vi "Test Panel - Add test (SubVI).vi"(8 "error in":errorcluster) -> (0 "error Out":errorcluster, 1 "Station":string, 2 "Cancel?":bool, 3 "Test Plan":string)   [LabVIEW 2019]
uses:
  Controls/Add test-state.ctl
  Controls/eFGV States.ctl
  Controls/FGV States.ctl
panel:
  in  "Path":path
  out "Station Data":string[](array[string])
  out "Status out":string[](array[string])
  in  "Select Station":u16(ring) items=["Please Select...", "TEST", "CONSOL", "UCT", "ISO CONS", "SATURATION", "TRIAXIALSHEAR", "TEST UU"]
  out "Select Test Plan form the list :":u16(ring) items=["Please Select...", "1dconsol.gs", "a", "abc.gs", "bcheck50.gs", "consol test.gs", "consol400-100.gs", "load12N(Table).gs", "load192N(Table).gs", "load24N(Table).gs", "load384N(Table).gs", "load48N(Table).gs", "load6N(Table).gs", "load96N(Table).gs", "loading12N.gs", "loading200N.gs", "loading24N.gs", "loading400N.gs", "loading48N.gs", "loading96N.gs", "sada.gs", "Sat100-90.gs", "Sat200-190.gs", "Sat300-290.gs", "Sat400-390.gs", "Sat50-40.gs", "Shearbox.gs", "test UU.gs", "test.gs", "test1.gs", "triaxialshear.gs", "uctcompressiontest.gs", "unload24(Table).gs", "unload24.gs", "unload96(Table).gs", "unload96.gs"]
  in  "OK":bool
  in  "Cancel":bool
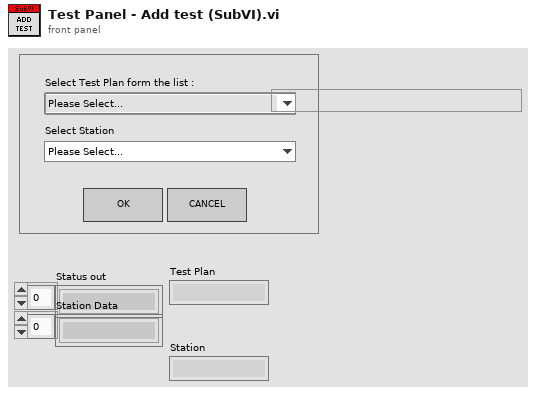
[diagram p1: front panel]
types:
  T1 = typedef "Add test-state.ctl" = enum16{"Init", "Idle", "Add", "Load Station", "Load", "Check Device", "Close", "Exit"}
  T2 = enum8{"Enabled", "Disabled", "Disabled and Grayed Out"}
  T3 = typedef "eFGV States.ctl" = enum16{"Init", "Read", "Write", "Exit"}
  T4 = typedef "FGV States.ctl" = enum16{"Read", "Write"}
  T5 = cluster{"TestPlan Section":string, "Key Value":string[]}[]
  T6 = cluster{"TestPlan Section":string, "Key Value":string[]}
  T7 = cluster{"Station Name":string, "Key Value":string[], "Key Names":string[]}[]
  T8 = cluster{"Station Name":string, "Key Value":string[], "Key Names":string[]}
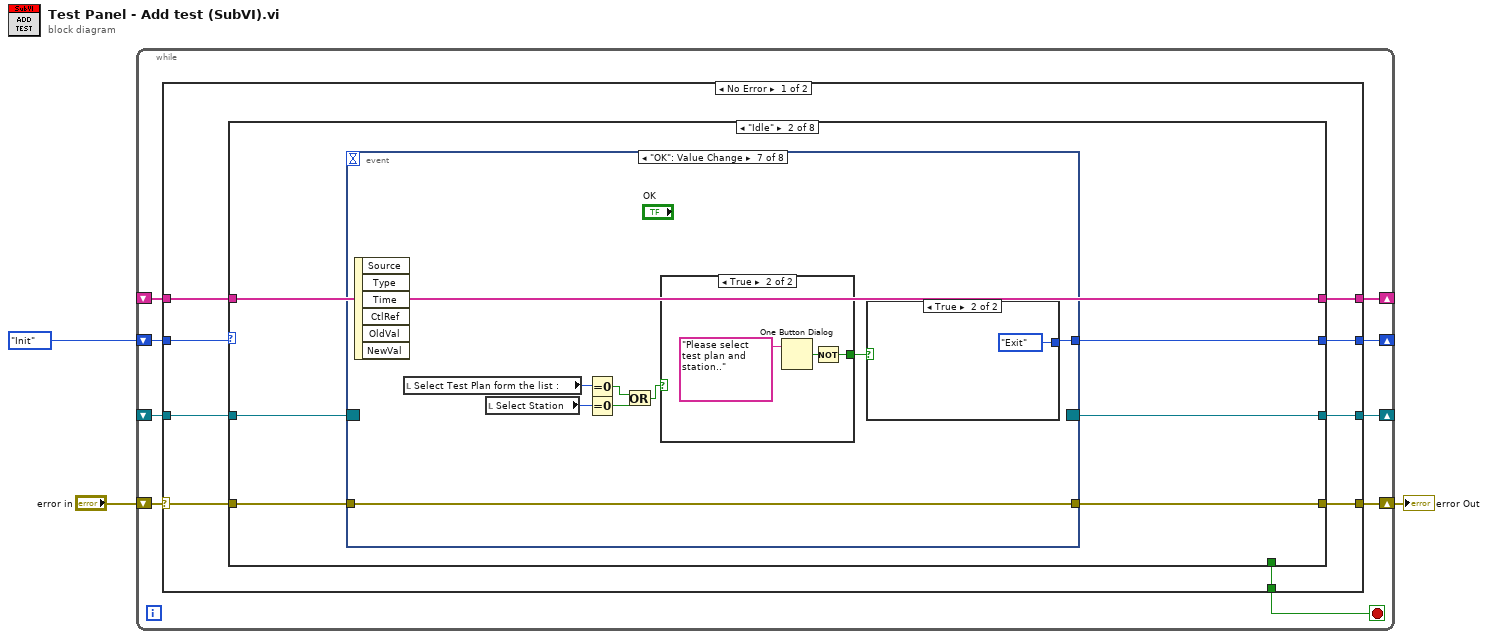
[diagram p0: block diagram]
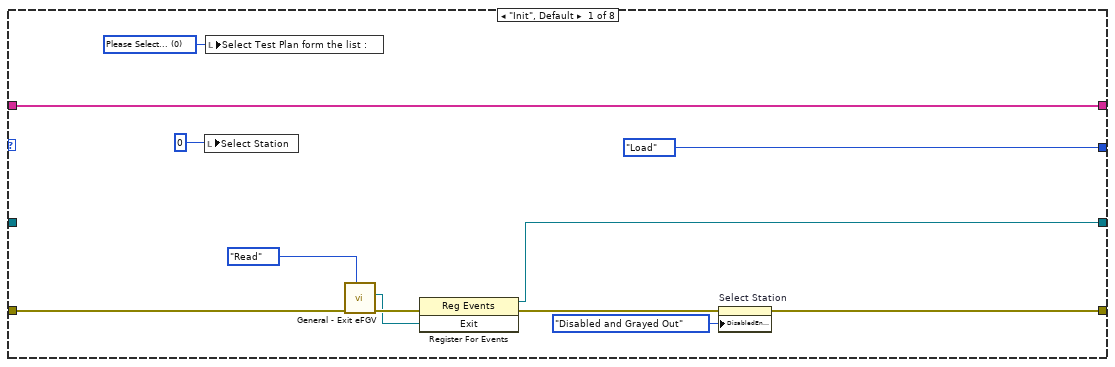
[diagram p2: hidden frame]
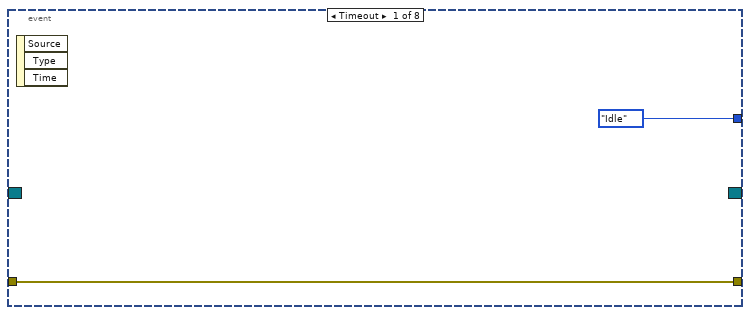
[diagram p3: hidden frame]
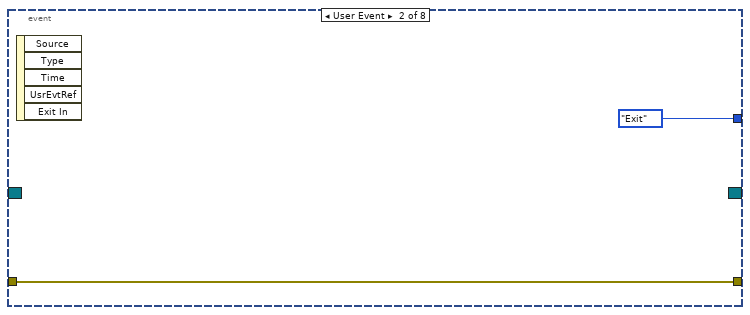
[diagram p4: hidden frame]
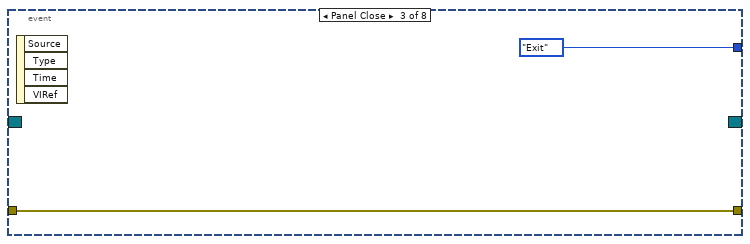
[diagram p5: hidden frame]
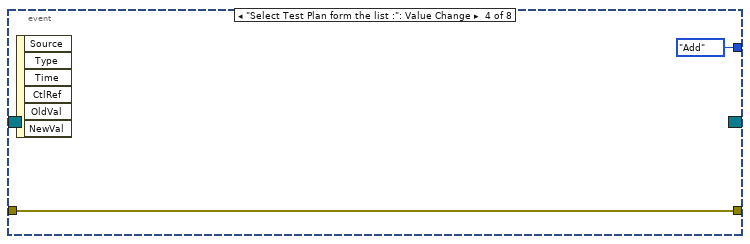
[diagram p6: hidden frame]
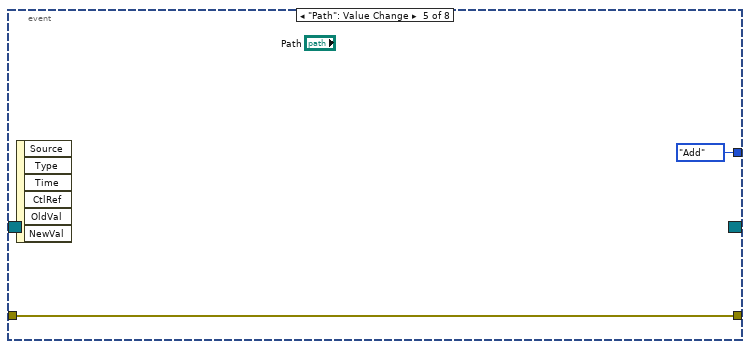
[diagram p7: hidden frame]
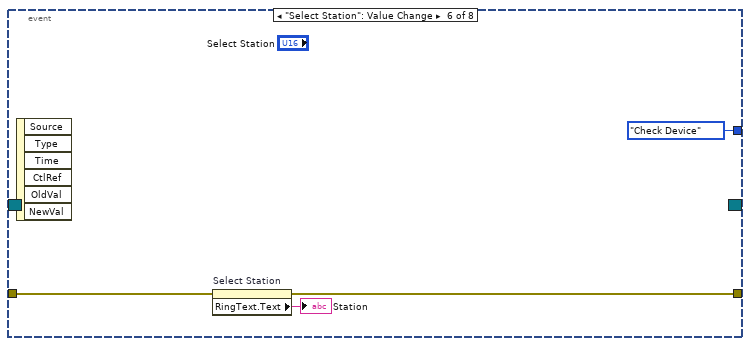
[diagram p8: hidden frame]
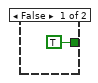
[diagram p9: hidden frame]
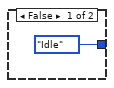
[diagram p10: hidden frame]
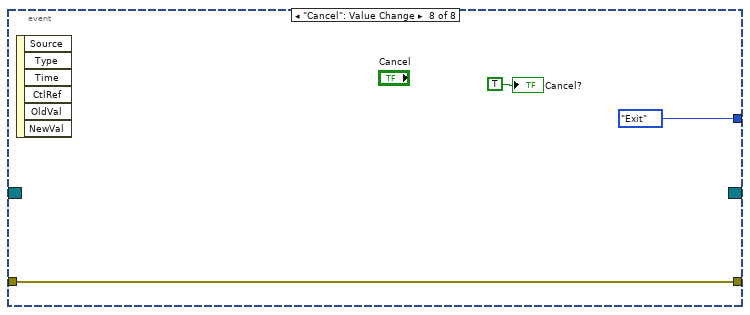
[diagram p11: hidden frame]
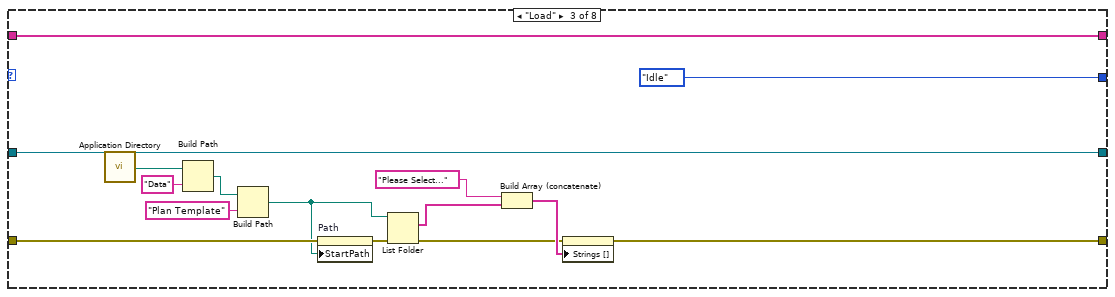
[diagram p12: hidden frame]
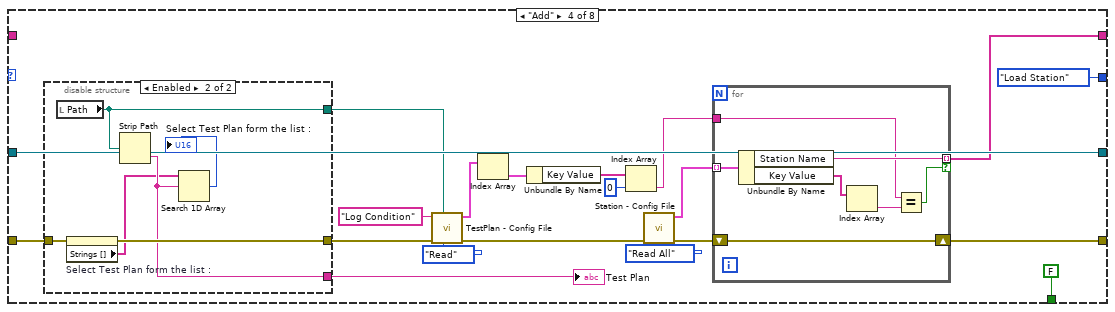
[diagram p13: hidden frame]
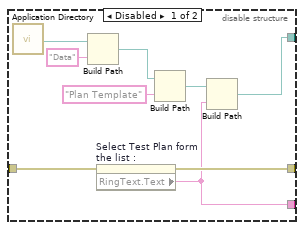
[diagram p14: hidden frame]
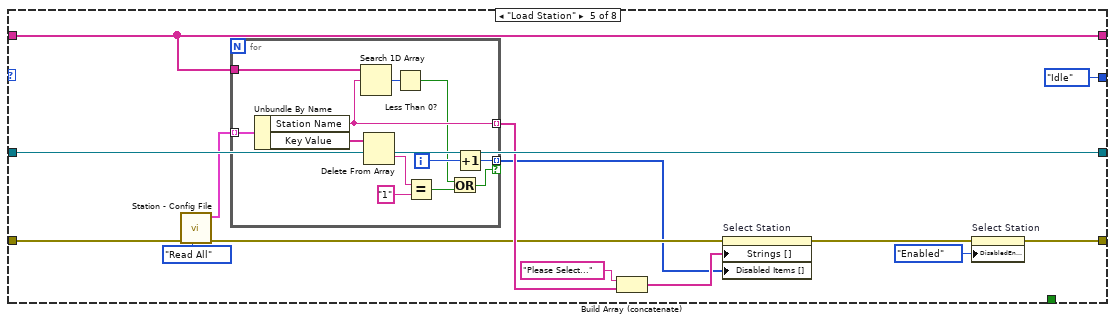
[diagram p15: hidden frame]
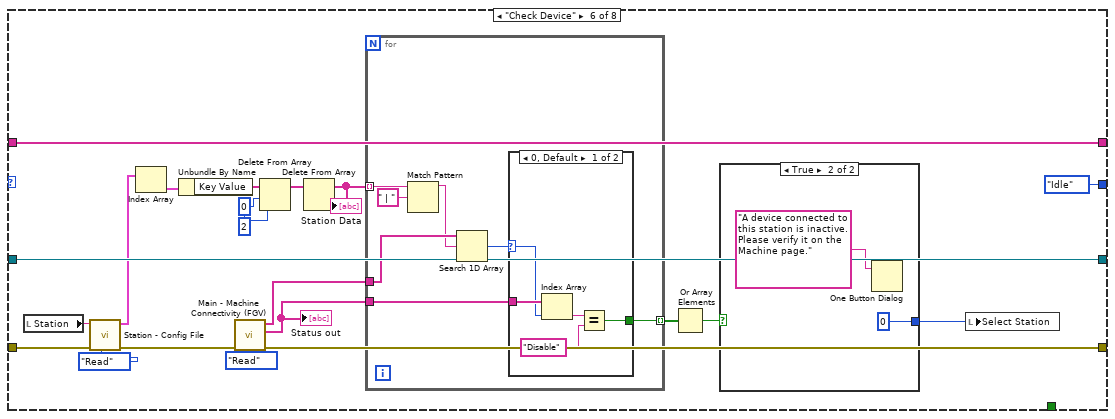
[diagram p16: hidden frame]
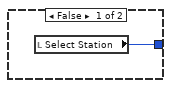
[diagram p17: hidden frame]
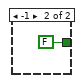
[diagram p18: hidden frame]
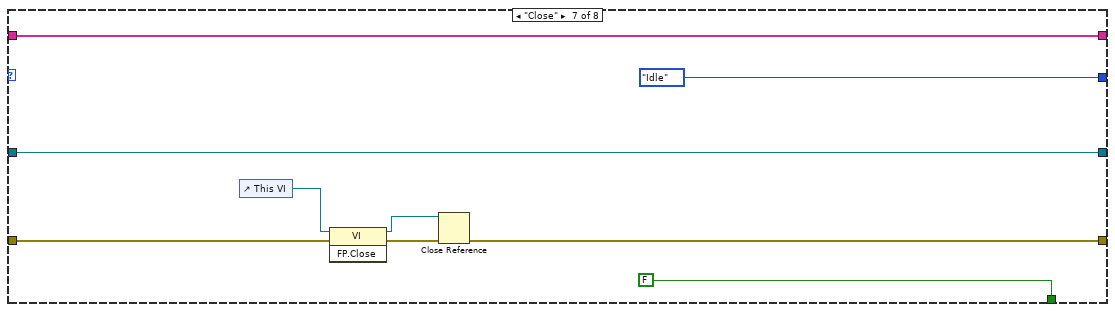
[diagram p19: hidden frame]
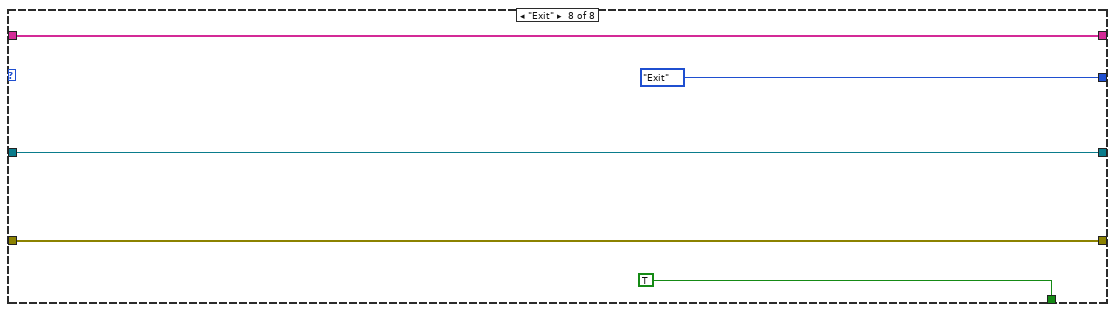
[diagram p20: hidden frame]
diagram:
  n1 = while {
    shift-right: [w11] -> w1
    shift-left: "error in" -> [w12]
    shift-right: [w9] -> _
    shift-left: Add_test-state."Init" -> [w10]
    shift-right: [w7] -> _
    shift-left: _ -> [w6]
    shift-right: [w5] -> _
    shift-left: _ -> [w4]
    stop <- w8 stop-if-true
    n2 = case shown="No Error" w12 {
      selector: w12 -> [w21 w210]
      tunnel: [w20 w208] -> w11
      tunnel: w10 -> [w19 _]
      tunnel: [w18 Add_test-state."Idle"] -> w9
      tunnel: [w17 _] -> w8
      tunnel: [w16 w209] -> w7
      tunnel: w6 -> [w15 w209]
      tunnel: [w14 w205] -> w5
      tunnel: w4 -> [w13 w205]
      frame No Error {
        n3 = case shown="\"Idle\"" w19 {
          tunnel: w21 -> [w29 w39 w72 w102 w136 w161 w195 w204]
          tunnel: [w24 w38 w74 w89 w128 w162 w193 w204] -> w20
          tunnel: [Add_test-state."Load" w37 Add_test-state."Idle" Add_test-state."Load Station" Add_test-state."Idle" Add_test-state."Idle" Add_test-state."Idle" Add_test-state."Exit"] -> w18
          tunnel: [_ _ _ FALSE _ _ FALSE TRUE] -> w17
          tunnel: [w30 w35 w85 w103 w141 w174 w199 w203] -> w16
          tunnel: w15 -> [_ w36 w85 w103 w141 w174 w199 w203]
          tunnel: [w26 w34 w75 w87 w131 w173 w191 w200] -> w14
          tunnel: w13 -> [w26 w34 w75 _ w131 w173 w191 w200]
          frame "Init", Default {
            w27 = u16 0 items=["Please Select..."] ("Select Test Plan form the list :")
            n4 = local write "Select Station"(0) -> ()
            n5 = local write "Select Test Plan form the list :"(w27) -> ()
            n6 = call "General - Exit eFGV.vi"("eFGV States"=eFGV_States."Read", "error in (no error)"=w29) -> ("error out"=w32:errorcluster, "Exit"=w31:refnum<user-event>)  [unwired: 7 in, 1 out]
            n7 = register-events(error in=w32, w31) -> (reference out=w30:refnum<event-registration>, error out=w25:errorcluster)  [unwired: 1 in]
            n8 = property on="Select Station" class="Ring (strict)"(error in=w25, "DisabledEnum"=T2."Disabled and Grayed Out" ("Disabled")) -> (error out=w24:errorcluster)  [unwired: 1 in, 1 out]
          }
          frame "Idle" {
            n9 = event shown="[6] \"OK\": Value Change" {
              selector: w36 -> [_ _ _ _ _ _ _ _]
              dyn-events: [_ _ _ _ _ _ _ _] -> w35
              timeout: _ -> [_ _ _ _ _ _ _ _]
              tunnel: w39 -> [w41 w43 w45 w47 w49 w51 w61 w69]
              tunnel: [w41 w43 w45 w47 w49 w52 w61 w69] -> w38
              tunnel: [Add_test-state."Idle" Add_test-state."Exit" Add_test-state."Exit" Add_test-state."Add" Add_test-state."Add" Add_test-state."Check Device" w59 Add_test-state."Exit"] -> w37
              event Timeout {
                n10 = event-data() -> ()  [unwired: 1 in, 3 out]
              }
              event User Event {
                n11 = event-data() -> ()  [unwired: 1 in, 5 out]
              }
              event Panel Close {
                n12 = event-data() -> ()  [unwired: 1 in, 4 out]
              }
              event "Select Test Plan form the list :": Value Change {
                n13 = event-data() -> ()  [unwired: 1 in, 6 out]
              }
              event "Path": Value Change {
                n14 = event-data() -> ()  [unwired: 1 in, 6 out]
              }
              event "Select Station": Value Change {
                n15 = event-data() -> ()  [unwired: 1 in, 6 out]
                n16 = property on="Select Station" class="Ring (strict)"(error in=w51) -> (error out=w52:errorcluster, "RingText.Text"=→"Station":string)  [unwired: 1 in, 1 out]
              }
              event "OK": Value Change {
                n17 = event-data() -> ()  [unwired: 1 in, 6 out]
                n18 = local read "Select Test Plan form the list :"() -> (w58:u16)
                n19 = local read "Select Station"() -> (w57:u16)
                n20 = Equal To 0?(x=w58) -> (x = 0?=w56:bool)
                n21 = Equal To 0?(x=w57) -> (x = 0?=w55:bool)
                n22 = Or(x=w56, y=w55) -> (x .or. y?=w54:bool)
                n23 = case shown="True" w54 {
                  tunnel: [TRUE w64] -> w60
                  frame False {
                  }
                  frame True {
                    n24 = One Button Dialog(message="Please select test plan and station..") -> (true=w65:bool)  [unwired: 1 in]
                    n25 = Not(x=w65) -> (.not. x?=w64:bool)
                  }
                }
                n26 = case shown="True" w60 {
                  tunnel: [Add_test-state."Idle" Add_test-state."Exit"] -> w59
                  frame False {
                  }
                  frame True {
                  }
                }
              }
              event "Cancel": Value Change {
                n27 = event-data() -> ()  [unwired: 1 in, 6 out]
                "Cancel?" <- TRUE
              }
            }
          }
          frame "Load" {
            n28 = call <vilib>:"Application Directory.vi"() -> ("Application Directory"=w77:path)
            n29 = Build Path(base path=w77, name or relative path="Data") -> (appended path=w76:path)
            n30 = Build Path(base path=w76, name or relative path="Plan Template") -> (appended path=w71:path)
            n31 = property on="Path" class="Path"(error in=w72, "StartPath"=w71) -> (error out=w73:errorcluster)  [unwired: 1 in, 1 out]
            n32 = List Folder(path=w71, error in=w73) -> (filenames=w79:string[], error out=w80:errorcluster)  [unwired: 2 in, 2 out]
            n33 = Build Array (concatenate)("Please Select...", w79) -> (w82:string[])
            n34 = property on="Select Test Plan form the list :" class="Ring (strict)"(error in=w80, "Strings []"=w82) -> (error out=w74:errorcluster)  [unwired: 1 in, 1 out]
          }
          frame "Add" {
            n35 = disable-structure shown="Enabled" {
              disable-tunnel: w102 -> [w114 w119]
              disable-tunnel: [w108 w118] -> w90
              disable-tunnel: [w107 w117] -> w88
              disable-tunnel: [w106 w120] -> w86
              frame Disabled {
                n36 = call <vilib>:"Application Directory.vi"() -> ("Application Directory"=w112:path)
                n37 = Build Path(base path=w112, name or relative path="Data") -> (appended path=w111:path)
                n38 = property on="Select Test Plan form the list :" class="Ring (strict)"(error in=w114) -> (error out=w108:errorcluster, "RingText.Text"=w107:string)  [unwired: 1 in, 1 out]
                n39 = Build Path(base path=w111, name or relative path="Plan Template") -> (appended path=w113:path)
                n40 = Build Path(base path=w113, name or relative path=w107) -> (appended path=w106:path)
              }
              frame Enabled {
                n41 = local read "Path"() -> (w120:path)
                n42 = property on="Select Test Plan form the list :" class="Ring (strict)"(error in=w119) -> (error out=w118:errorcluster, "Strings []"=w116:string[])  [unwired: 1 in, 1 out]
                n43 = Strip Path(path=w120) -> (name=w117:string)  [unwired: 1 out]
                n44 = Search 1D Array(1D array=w116, element=w117) -> (index of element=→"Select Test Plan form the list :":i32)  [unwired: 1 in]
              }
            }
            "Test Plan" <- w88
            n45 = call "TestPlan - Config File.vi"("Action"=enum16{"Write", "Read", "Read All", "Remove"}."Read", "file path"=w86, "error in (no error)"=w90, "TestPlan Section"="Log Condition") -> ("error out"=w98:errorcluster, "Value Out"=w96:T5)  [unwired: 5 in, 1 out]
            n46 = Index Array(array=w96) -> (element=w95:T6)  [unwired: 1 in]
            n47 = Unbundle By Name(w95) -> ("Key Value"=w97:string[])
            n48 = Index Array(array=w97, index=0) -> (element=w101:string)
            n49 = call "Station - Config File.vi"("Action"=enum16{"Write", "Read", "Read All", "Remove"}."Read All", "error in (no error)"=w98) -> ("error out"=w100:errorcluster, "Value Out"=w99:T7)  [unwired: 8 in]
            n50 = for {
              tunnel: w99 -> [w127] mode=indexing
              tunnel: [w125] -> w87 mode=indexing if=w121
              tunnel: w101 -> [w122]
              shift-right: [w124] -> w89
              shift-left: w100 -> [w124]
              n51 = Unbundle By Name(w127) -> ("Station Name"=w125:string, "Key Value"=w126:string[])
              n52 = Index Array(array=w126) -> (element=w123:string)  [unwired: 1 in]
              n53 = Equal?(x=w122, y=w123) -> (x = y?=w121:bool)
            }
          }
          frame "Load Station" {
            n54 = call "Station - Config File.vi"("Action"=enum16{"Write", "Read", "Read All", "Remove"}."Read All", "error in (no error)"=w136) -> ("error out"=w135:errorcluster, "Value Out"=w138:T7)  [unwired: 8 in]
            n55 = for {
              tunnel: w138 -> [w153] mode=indexing
              tunnel: [w146] -> w137 mode=indexing
              tunnel: [w150] -> w133 mode=indexing if=w142
              tunnel: w131 -> [w147]
              i -> [w151]
              n56 = Unbundle By Name(w153) -> ("Station Name"=w146:string, "Key Value"=w152:string[])
              n57 = Search 1D Array(1D array=w147, element=w146) -> (index of element=w145:i32)  [unwired: 1 in]
              n58 = Delete From Array(array=w152) -> (deleted portion=w149:string)  [unwired: 2 in, 1 out]
              n59 = Less Than 0?(x=w145) -> (x < 0?=w143:bool)
              n60 = Equal?(x=w149, y="1") -> (x = y?=w144:bool)
              n61 = Or(x=w143, y=w144) -> (x .or. y?=w142:bool)
              n62 = Increment(x=w151) -> (x+1=w150:i32)
            }
            n63 = Build Array (concatenate)("Please Select..." ("String"), w137) -> (w134:string[])
            n64 = property on="Select Station" class="Ring (strict)"(error in=w135, "Strings []"=w134, "Disabled Items []"=w133) -> (error out=w129:errorcluster)  [unwired: 1 in, 1 out]
            n65 = property on="Select Station" class="Ring (strict)"(error in=w129, "DisabledEnum"=T2."Enabled" ("Disabled")) -> (error out=w128:errorcluster)  [unwired: 1 in, 1 out]
          }
          frame "Check Device" {
            n66 = local read "Station"() -> (w160:string)
            n67 = call "Station - Config File.vi"("Action"=enum16{"Write", "Read", "Read All", "Remove"}."Read", "error in (no error)"=w161, "Station Name"=w160) -> ("error out"=w167:errorcluster, "Value Out"=w168:T7)  [unwired: 7 in]
            n68 = Index Array(array=w168) -> (element=w169:T8)  [unwired: 1 in]
            n69 = Unbundle By Name(w169) -> ("Key Value"=w171:string[])
            n70 = call "Main - Machine Connectivity (FGV).vi"("Action"=FGV_States."Read", "error In"=w167) -> ("error out"=w162:errorcluster, "Status out"=w157:string[], "Device Name out"=w158:string[])  [unwired: 7 in]
            "Status out" <- w157
            n71 = Delete From Array(array=w171, length=2, index=0) -> (array with subset deleted=w170:string[])  [unwired: 1 out]
            n72 = Delete From Array(array=w170) -> (array with subset deleted=w159:string[])  [unwired: 2 in, 1 out]
            "Station Data" <- w159
            n73 = for {
              tunnel: w159 -> [w183] mode=indexing
              tunnel: w158 -> [w182]
              tunnel: w157 -> [w180]
              tunnel: [w178] -> w156 mode=indexing
              n74 = Match Pattern(string=w183, regular expression=" | ") -> (before substring=w181:string)  [unwired: 1 in, 3 out]
              n75 = Search 1D Array(1D array=w182, element=w181) -> (index of element=w179:i32)  [unwired: 1 in]
              n76 = case shown="0, Default" w179 {
                selector: w179 -> [w188 _]
                tunnel: w180 -> [w189 _]
                tunnel: [w185 FALSE] -> w178
                frame 0, Default {
                  n77 = Index Array(array=w189, index=w188) -> (element=w187:string)
                  n78 = Equal?(x=w187, y="Disable") -> (x = y?=w185:bool)
                }
                frame -1 {
                }
              }
            }
            n79 = Or Array Elements(Boolean array=w156) -> (logical OR=w155:bool)
            n80 = case shown="True" w155 {
              tunnel: [w175 u16 0] -> w154
              frame False {
                n81 = local read "Select Station"() -> (w175:u16)
              }
              frame True {
                n82 = One Button Dialog(message="A device connected to this station is inactive. Please verify it on the Machine page.") -> ()  [unwired: 1 in, 1 out]
              }
            }
            n83 = local write "Select Station"(w154) -> ()
          }
          frame "Close" {
            n84 = control-ref of="This VI"() -> (w194:refnum<vi>)
            n85 = invoke class="VI" method="FP.Close"(reference=w194, error in=w195) -> (reference out=w192:refnum<vi>, error out=w196:errorcluster)  [unwired: 1 in, 1 out]
            n86 = Close Reference(reference=w192, error in (no error)=w196) -> (error out=w193:errorcluster)
          }
          frame "Exit" {
          }
        }
      }
      frame Error {
        n87 = call <vilib>:"Clear Errors.vi"("error in (no error)"=w210) -> ("error out"=w208:errorcluster)  [unwired: 5 in, 1 out]
        n88 = Wait (ms)(milliseconds to wait=u32 100) -> ()  [unwired: 1 out]
      }
    }
  }
  "error Out" <- w1
